vi "InitialVIMarcoGonzalez.vi"() -> ()   [LabVIEW 2012]
panel:
  in  "Threshold C":dbl
  in  "Threshold F":dbl
  out "?":bool
  out "?":bool
  in  "?":bool
  out "Celsius":dbl
  out "Fahrenheit":dbl
  in  "Fahrenheit":dbl
  in  "Celsius":dbl
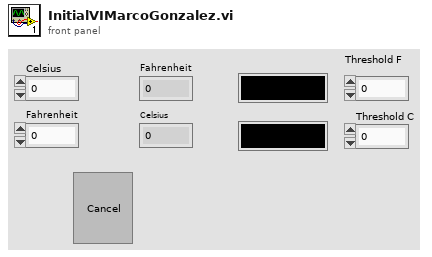
[diagram p1: front panel]
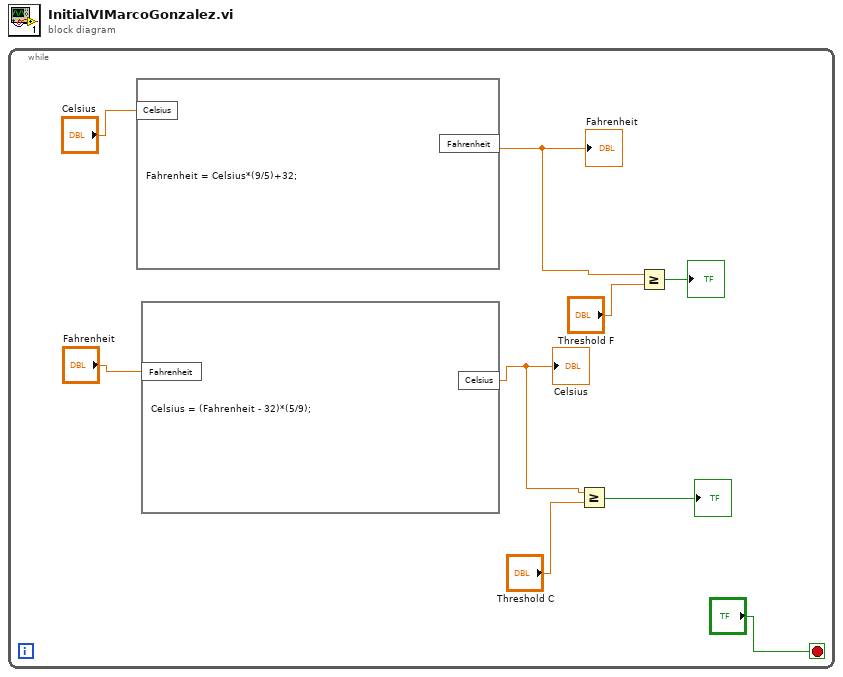
[diagram p0: block diagram]
diagram:
  n1 = while {
    stop <- "?" stop-if-true
    n2 = formula code="Fahrenheit = Celsius*(9/5)+32;"("Celsius"="Celsius") -> ("Fahrenheit"=w5:dbl)
    "Fahrenheit" <- w5
    n3 = formula code="Celsius = (Fahrenheit - 32)*(5/9);"("Fahrenheit"="Fahrenheit") -> ("Celsius"=w7:dbl)
    "Celsius" <- w7
    n4 = Greater Or Equal?(x=w7, y="Threshold C") -> (x >= y?=→"?":bool)
    n5 = Greater Or Equal?(x=w5, y="Threshold F") -> (x >= y?=→"?":bool)
  }
